vi "emi_CRC 16 CCITT.vi"(7 "Raw data":u8[](array[numeric])) -> (8 "CCITT crc 16":u16, 10 "CCITT crc 16 bytes":u8[](array[numeric]))   [LabVIEW 2011]
doc: "Calculate the CCITT CRC 16 from an array of u8. \n\nInitial Value: FFFF\nPolynomial: x16 + x12 + x5 + 1ss\n\nSubroutine reentrant for throughput"
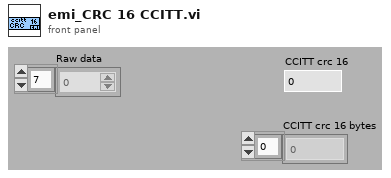
[diagram p1: front panel]
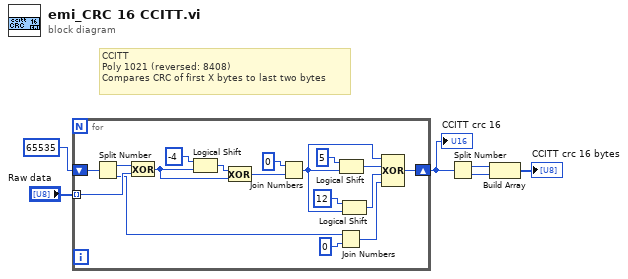
[diagram p0: block diagram]
diagram:
  # "CCITT\nPoly 1021 (reversed: 8408)\nCompares CRC of first X bytes to last two bytes"
  n1 = for {
    tunnel: "Raw data" -> [w17] mode=indexing
    shift-right: [w7] -> w2
    shift-left: u16 65535 -> [w16]
    n2 = Split Number(x=w16) -> (hi(x)=w23:u8, lo(x)=w10:u8)
    n3 = Exclusive Or(1:w17, 2:w23) -> (0:w20:u8)
    n4 = Logical Shift(y=i8 -4, x=w20) -> (x << y=w21:u8)
    n5 = Exclusive Or(1:w20, 2:w21) -> (0:w19:u8)
    n6 = Join Numbers(hi=u8 0, lo=w19) -> ((hi.lo)=w12:u16)
    n7 = Logical Shift(y=i8 5, x=w12) -> (x << y=w14:u16)
    n8 = Join Numbers(hi=w10, lo=u8 0) -> ((hi.lo)=w8:u16)
    n9 = Logical Shift(y=i8 12, x=w12) -> (x << y=w11:u16)
    n10 = Compound Arithmetic op=XOR(w12, w14, w11, w8) -> (w7:u16)
  }
  "CCITT crc 16" <- w2
  n11 = Split Number(x=w2) -> (hi(x)=w6:u8, lo(x)=w5:u8)
  n12 = Build Array(w6, w5) -> (→"CCITT crc 16 bytes":u8[])
